vi "4-Rotina de processamento dos dados de calibração.vi"() -> ()   [LabVIEW 2018]
uses:
  <vilib>/Analysis/baseanly.llb/Mean (DBL).vi
  <vilib>/Analysis/NI_AALBase.lvlib
panel:
  out "Erro Relativo da Calibração":dbl[](array[numeric]) format="%#.4g"
  out "Sinal de Força em tempo real":dbl[](graph)
  out "XY Graph":cluster{"Y":dbl[], "Y":dbl[]}[](graph)
  out "Carga Experimental (N)":dbl[](array[numeric]) format="%#.2g"
  out "Carga Calculada - valores médios (N)":dbl[](array[numeric]) format="%#.2g"
  # "PROGRAMA DE PROCESSAMENTO DOS DADOS DE CALIBRAÇÃO"
  # "Força Aplicada (N):"
  # "Força Medida (N):"
  # "Erro Relativo (N):"
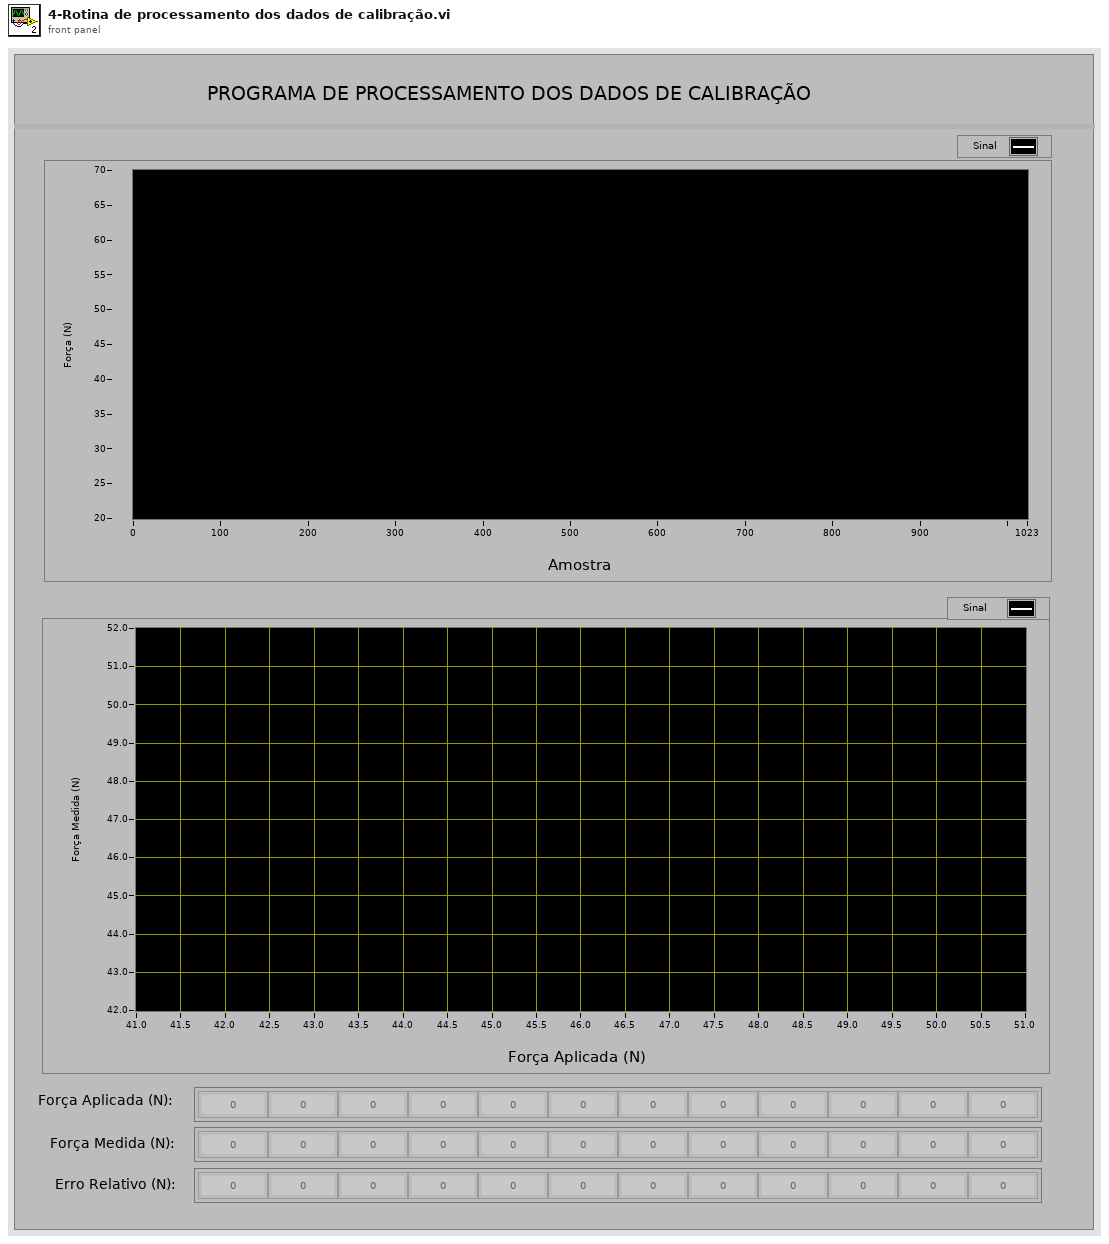
[diagram p1: front panel]
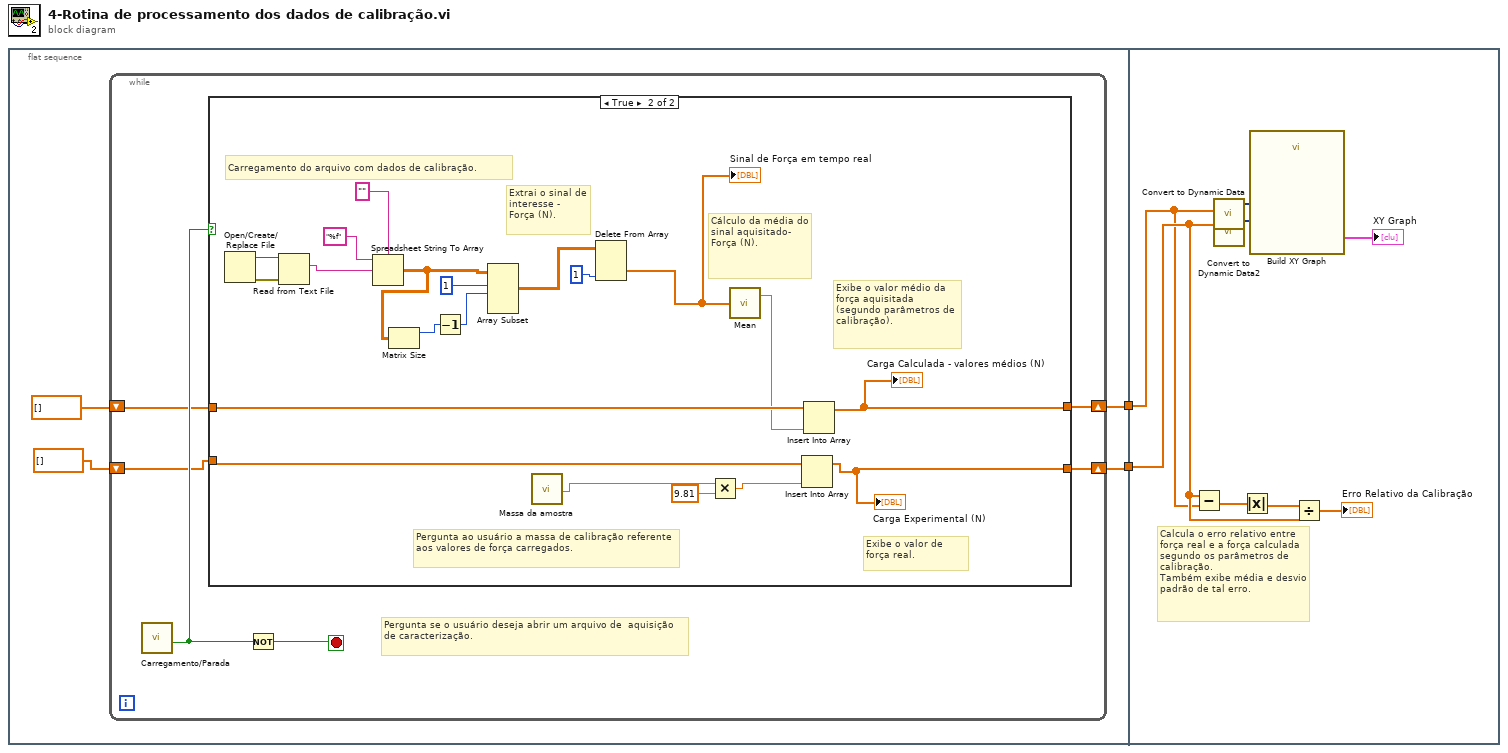
[diagram p0: block diagram]
diagram:
  n1 = flat-sequence {
    tunnel: [w5] -> w2
    tunnel: [w3] -> w1
    tunnel: w2 -> [w35]
    tunnel: w1 -> [w37]
    frame #0 {
      n2 = while {
        shift-right: [w9] -> w5
        shift-left: dbl[] [] ("array") -> [w10]
        shift-right: [w7] -> w3
        shift-left: dbl[] [] ("array") -> [w8]
        stop <- w12 stop-if-true
        # "Pergunta se o usuário deseja abrir um arquivo de  aquisição de caracterização."
        n3 = call "Carregamento/Parada"() -> ("Carregar"=w11:bool)  [unwired: 18 in, 1 out]
        n4 = case shown="True" w11 {
          tunnel: w10 -> [w14 w30]
          tunnel: [w14 w26] -> w9
          tunnel: w8 -> [w13 w29]
          tunnel: [w13 w27] -> w7
          frame False {
          }
          frame True {
            # "Exibe o valor de força real."
            # "Exibe o valor médio da força aquisitada (segundo parâmetros de calibração)."
            # "Cálculo da média do sinal aquisitado-  Força (N)."
            # "Carregamento do arquivo com dados de calibração."
            # "Pergunta ao usuário a massa de calibração referente aos valores de força carregados."
            # "Extrai o sinal de interesse - Força (N)."
            n5 = Open/Create/Replace File() -> (refnum out=w34:refnum<file>, error out=w32:errorcluster)  [unwired: 6 in, 1 out]
            n6 = Read from Text File(file (use dialog)=w34, error in=w32) -> (text=w31:string)  [unwired: 2 in, 3 out]
            n7 = Spreadsheet String To Array(delimiter (Tab)="", format string="%f", spreadsheet string=w31) -> (array=w20:dbl[][])  [unwired: 1 in]
            n8 = Matrix Size(0:w20) -> (1:w22:i32)  [unwired: 1 out]
            n9 = Decrement(x=w22) -> (x-1=w21:i32)
            n10 = Array Subset(array=w20, index (row)=1 ("row 1"), length (row)=w21) -> (w23:dbl[][])  [unwired: 2 in]
            n11 = call "Massa da amostra"() -> ("Massa"=w19:dbl)  [unwired: 17 in, 2 out]
            n12 = Delete From Array(array=w23, index (col)=1 ("disabled index (col)")) -> (deleted portion=w15:dbl[])  [unwired: 2 in, 1 out]
            "Sinal de Força em tempo real" <- w15
            n13 = Multiply(x=w19, y=9.81) -> (x*y=w17:dbl)
            n14 = call-poly <vilib>:"Mean.vi"("X"=w15) -> ("mean"=w28:dbl)  [unwired: 1 out]
            n15 = Insert Into Array(array=w29, new element=w17) -> (w27:dbl[])  [unwired: 1 in]
            "Carga Experimental (N)" <- w27
            n16 = Insert Into Array(array=w30, new element=w28) -> (w26:dbl[])  [unwired: 1 in]
            "Carga Calculada - valores médios (N)" <- w26
          }
        }
        n17 = Not(x=w11) -> (.not. x?=w12:bool)
      }
    }
    frame #1 {
      # "Calcula o erro relativo entre força real e a força calculada segundo os parâmetros de calibração.\nTambém exibe média e desvio padrão de tal erro."
      n18 = Subtract(x=w37, y=w35) -> (x-y=w39:dbl[])
      n19 = call "Convert to Dynamic Data"("Array"=w37) -> ("Dynamic Data Type"=w41:dynamicdata)  [unwired: 3 in]
      n20 = call "Convert to Dynamic Data2"("Array"=w35) -> ("Dynamic Data Type"=w40:dynamicdata)  [unwired: 3 in]
      n21 = Absolute Value(x=w39) -> (abs(x)=w38:dbl[])
      n22 = call "Build XY Graph"("Y Input"=w40, "X Input"=w41) -> ("XY Graph"=→"XY Graph":cluster{"Y":dbl[], "Y":dbl[]}[])  [unwired: 3 in, 6 out]
      n23 = Divide(x=w38, y=w37) -> (x/y=→"Erro Relativo da Calibração":dbl[])
    }
  }
